vi "SetOutputWaveform.vi"(8 "error in (no error)":errorcluster, 10 "OutputWaveform.lvclass":refnum<class "OutputWaveform.lvclass">, 11 "FunctionGenerator in":refnum<class "FunctionGenerator.lvclass">) -> (0 "error out":errorcluster, 3 "FunctionGenerator out":refnum<class "FunctionGenerator.lvclass">)   [LabVIEW 2020, in "FunctionGenerator.lvclass"]
uses:
  FunctionGenerator.lvclass
  OutputWaveform/OutputWaveform.lvclass
  FunctionGenerator.lvclass/FunctionGenerator.ctl
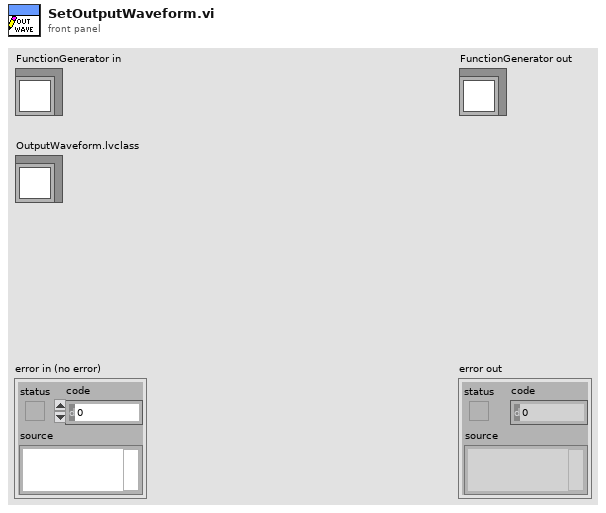
[diagram p1: front panel]
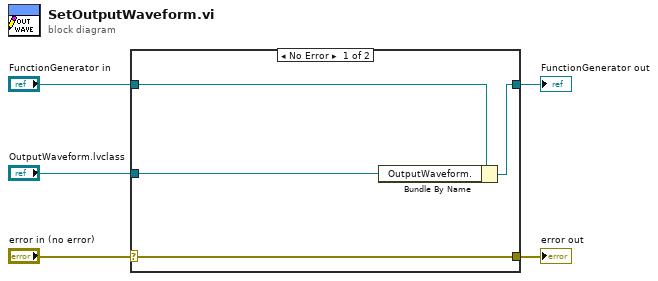
[diagram p0: block diagram]
diagram:
  n1 = case shown="No Error" "error in (no error)" {
    selector: "error in (no error)" -> [w9 w10]
    tunnel: [w9 w10] -> w4
    tunnel: [w7 w11] -> w2
    tunnel: "FunctionGenerator in" -> [w8 w11]
    tunnel: "OutputWaveform.lvclass" -> [w6 _]
    frame No Error {
      n2 = Bundle By Name(cluster=w8, "OutputWaveform."=w6) -> (w7:refnum<class "FunctionGenerator.lvclass">)
    }
    frame Error {
    }
  }
  "error out" <- w4
  "FunctionGenerator out" <- w2
